vi "Digital Handler.vi"(0 "Variable Index":i32, 1 "Action":T2, 5 "End Tid":dbl, 7 "Value":bool, 9 "Upd freq":T1, 11 "error in (no error)":errorcluster, 12 "Start tid(buff size":dbl) -> (3 "Indexes":i32[](array[numeric]), 6 "Value out":bool, 8 "Digital Waveform":digitalwaveform(waveform)={"t0"=timestamp(0 s since 1904-01-01), "dt"=1.0, "Y"={"transitions"=[], "data"=[]}}, 10 "Values":bool[](array[boolean]), 14 "Numb var":i32, 15 "error out":errorcluster)   [LabVIEW 2010]
uses:
  Action Analog Handler.ctl
  Update frequensies.ctl
  Digital Psudo WF.ctl
  <vilib>/Waveform/DTblOps.llb/DTbl Boolean Array to Digital.vi
panel:
  out "Time Stamp":timestamp
  # "OBS, \nBruk Value som oppdaterings frekvens \nunder reg new var."
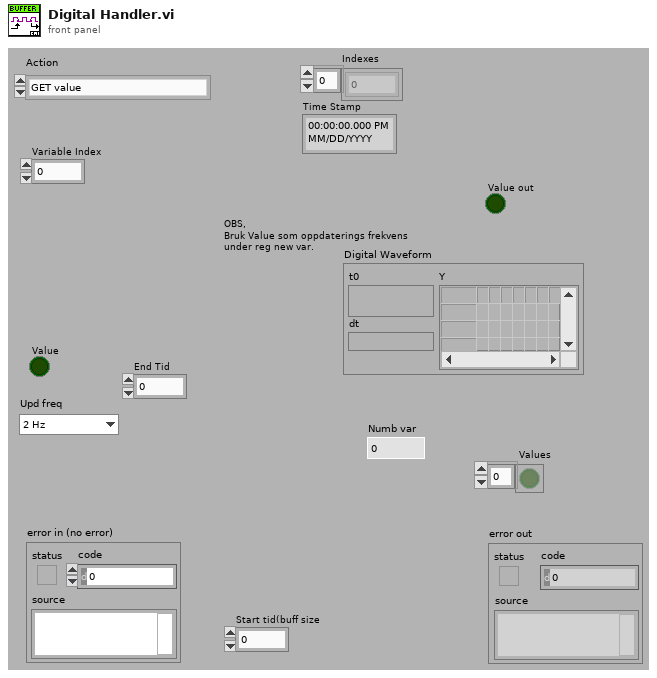
[diagram p1: front panel]
types:
  T1 = typedef "Update frequensies.ctl" = enum16{"2 Hz", "1 Hz", "0.1 Hz"}
  T2 = typedef "Action Analog Handler.ctl" = enum16{"GET value", "GET Single Frequenzy", "GET All Values", "GET Waveform", "Get Numb Var", "SET Value", "START Buffer", "REG Variable", "BUF size(total antal sekund)", "PULS", "Get a Value at time"}
  T3 = typedef "Digital Psudo WF.ctl" = cluster{"\ndata":bool[], "Index":i32, "Upd freq":T1, "Last index time":dbl, "Rounded":bool}
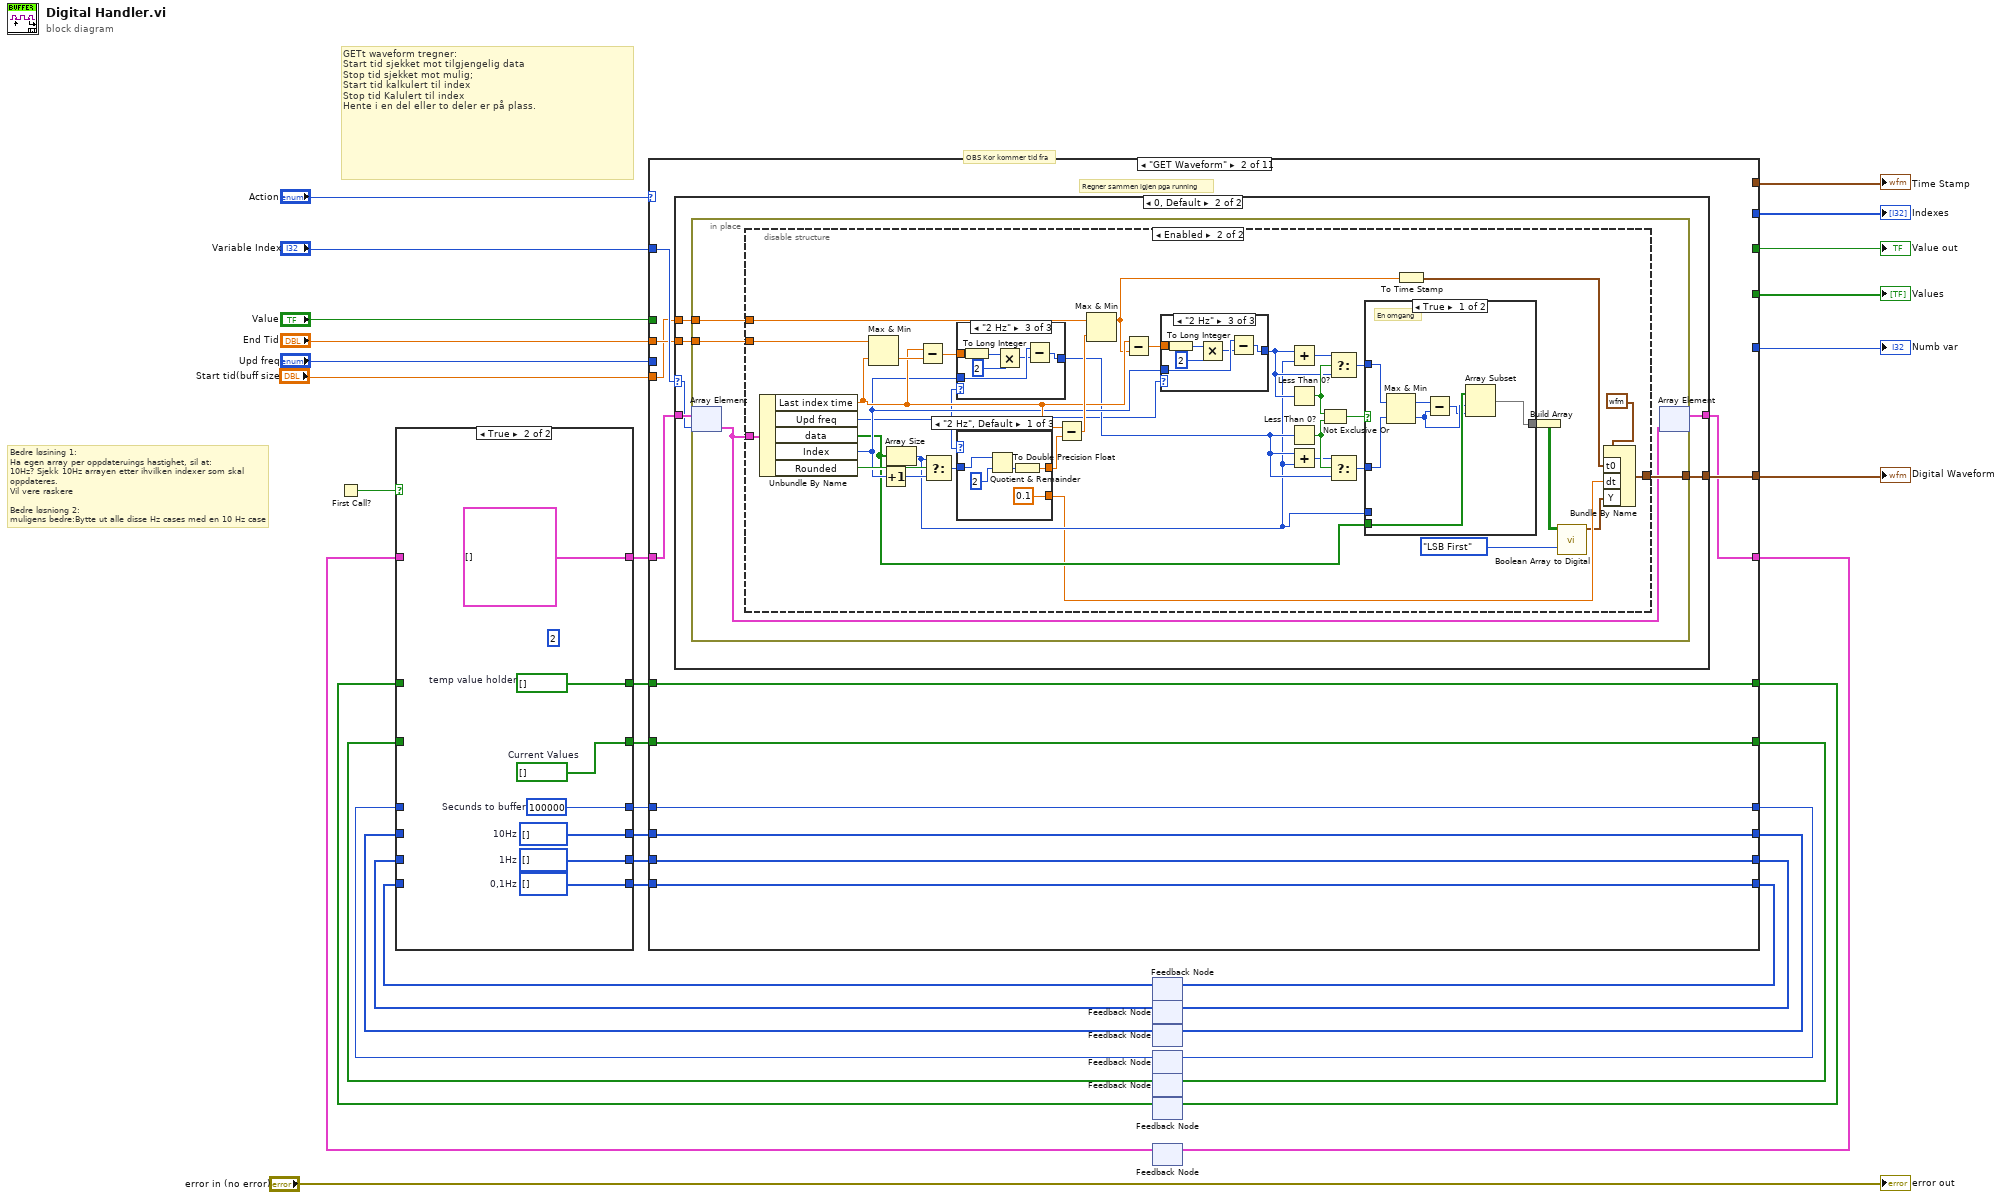
[diagram p0: block diagram]
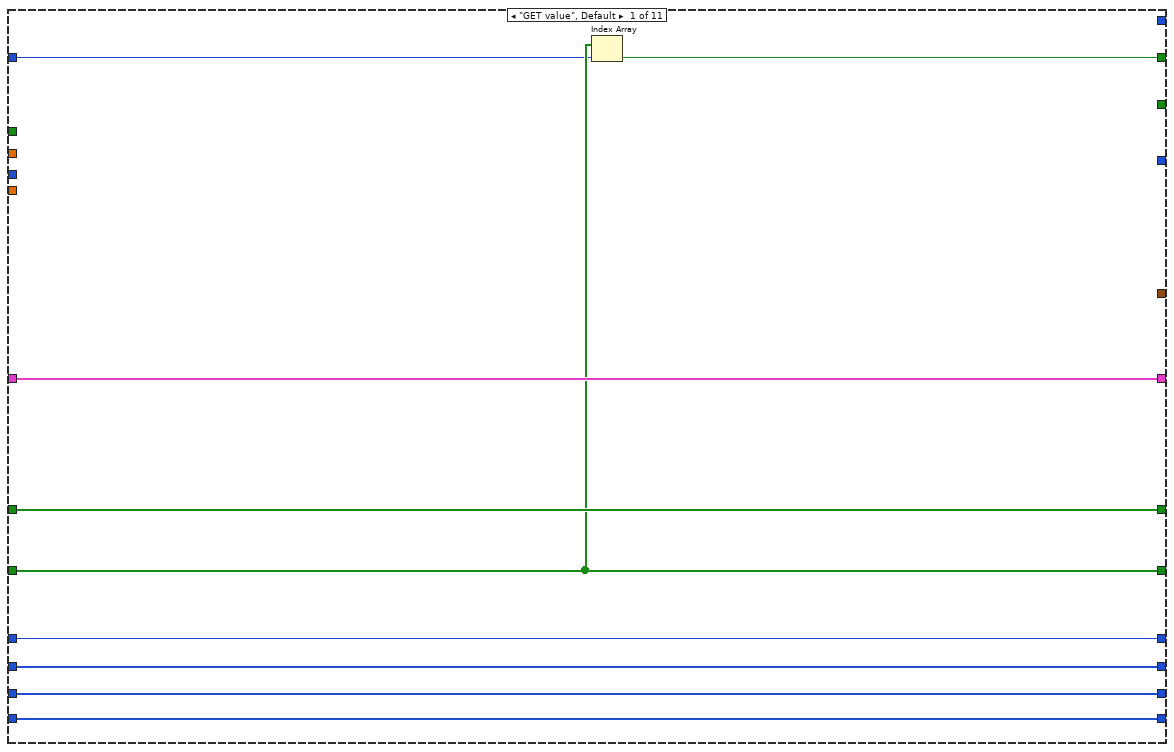
[diagram p3: hidden frame]
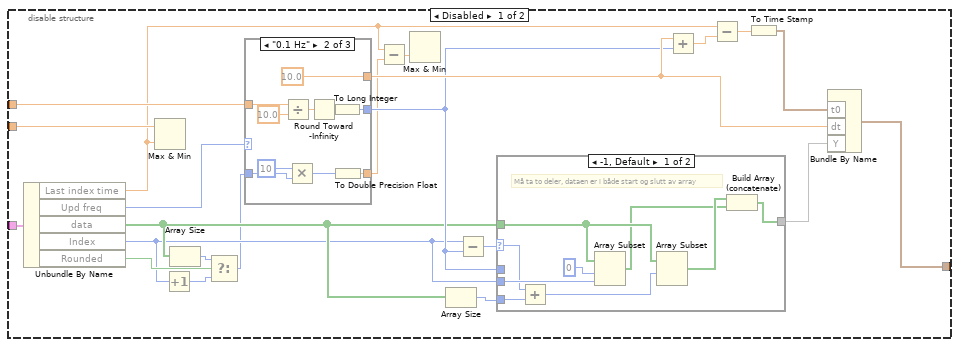
[diagram p5: hidden frame]
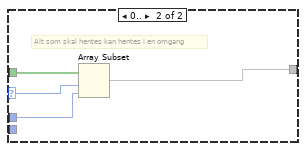
[diagram p6: hidden frame]
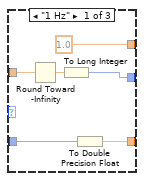
[diagram p7: hidden frame]
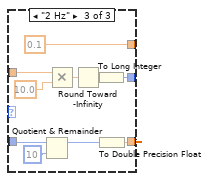
[diagram p8: hidden frame]
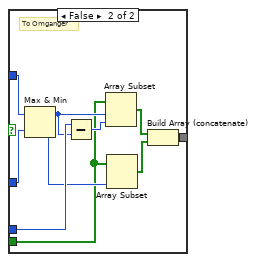
[diagram p9: hidden frame]
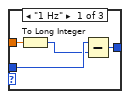
[diagram p10: hidden frame]
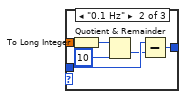
[diagram p11: hidden frame]
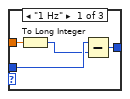
[diagram p12: hidden frame]
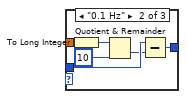
[diagram p13: hidden frame]
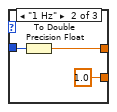
[diagram p14: hidden frame]
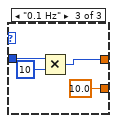
[diagram p15: hidden frame]
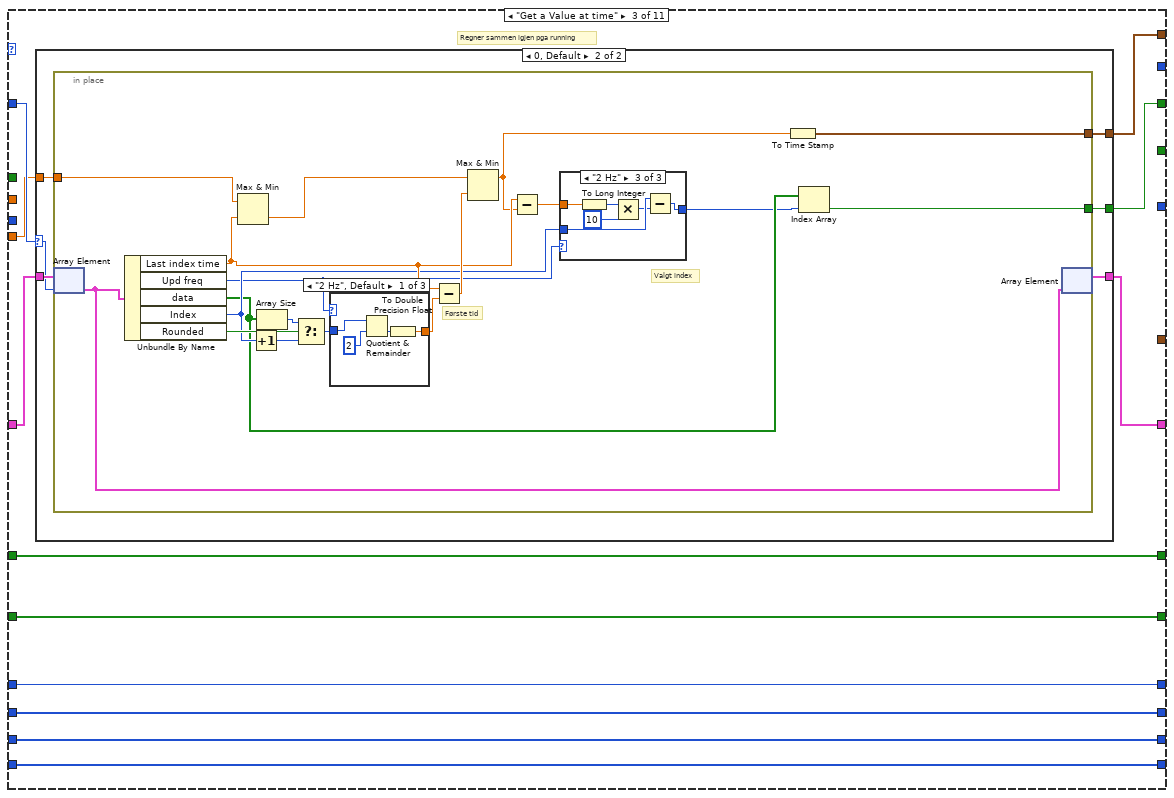
[diagram p16: hidden frame]
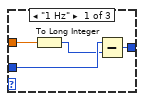
[diagram p18: hidden frame]
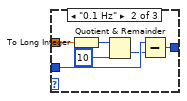
[diagram p19: hidden frame]
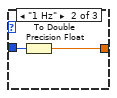
[diagram p20: hidden frame]
diagram:
  # "GETt waveform tregner:\nStart tid sjekket mot tilgjengelig data\nStop tid sjekket mot mulig;\nStart tid kalkulert til index\nStop tid Kalulert til index\nHente i en del eller to deler er på plass."
  # "OBS Kor kommer tid fra"
  # "Bedre løsining 1:\nHa egen array per oppdateruings hastighet, sil at:\n10Hz? Sjekk 10Hz arrayen etter ihvilken indexer som skal oppdateres.\nVil vere raskere\n\nBedre løsniong 2:\nmuligens bedre:Bytte ut alle disse Hz cases med en 10 Hz case"
  n1 = First Call?() -> (First Call?: T/F=w32:bool)
  n2 = feedback #1() -> (w9:i32[])  [unwired: 1 in]
  n3 = feedback #2() -> (w10:i32[])  [unwired: 1 in]
  n4 = feedback #3() -> (w11:i32[])  [unwired: 1 in]
  n5 = feedback #4() -> (w8:i32)  [unwired: 1 in]
  n6 = feedback #5() -> (w25:bool[])  [unwired: 1 in]
  n7 = feedback #6() -> (w26:bool[])  [unwired: 1 in]
  n8 = feedback #7() -> (w33:T3[])  [unwired: 1 in]
  n9 = case shown="True" w32 {
    tunnel: w33 -> [w42 _]
    tunnel: [w42 T3[] []] -> w2
    tunnel: [w41 w49] -> w30
    tunnel: [w40 w48] -> w29
    tunnel: w26 -> [w41 _]
    tunnel: w25 -> [w40 _]
    tunnel: [w36 w47] -> w23
    tunnel: [w39 w46] -> w17
    tunnel: [w38 w45] -> w14
    tunnel: [w37 w44] -> w12
    tunnel: w11 -> [w39 _]
    tunnel: w10 -> [w38 _]
    tunnel: w9 -> [w37 _]
    tunnel: w8 -> [w36 _]
    frame False {
    }
    frame True {
      (unwired) u8 2 ("ValDigital - Status value(0 F, 1 T, 2 NA)")
      w44 = i32[] []  # 0,1Hz
      w45 = i32[] []  # 1Hz
      w46 = i32[] []  # 10Hz
      w47 = 100000  # Secunds to buffer
      w48 = bool[] []  # Current Values
      w49 = bool[] []  # temp value holder
    }
  }
  n10 = case shown="\"GET Waveform\"" "Action" {
    tunnel: [w58 w62 w242 w307 w317 w326 w341 w388 w414 w442 w506] -> w31
    tunnel: w2 -> [w58 w63 w243 w307 w317 w326 w340 w388 w414 w447 w509]
    tunnel: w30 -> [w57 w70 w249 w300 w314 w325 w338 w389 w416 w424 w508]
    tunnel: w29 -> [w56 w69 w248 w306 w316 w324 w336 w395 w410 w443 w507]
    tunnel: [w57 w70 w249 w300 w313 w325 w339 w389 w416 w441 w505] -> w27
    tunnel: [w56 w69 w248 w306 w316 w324 w337 w396 w410 w440 w504] -> w28
    tunnel: [w53 w60 w241 w305 w315 w320 w335 w394 w415 w421 w510] -> w24
    tunnel: w23 -> [w53 w60 w241 w305 w315 _ w335 w394 w415 w421 w510]
    tunnel: "Variable Index" -> [w54 w64 w244 _ w311 _ _ _ _ w423 w503]
    tunnel: "Value" -> [_ _ _ _ w312 _ _ _ _ _ _]
    tunnel: [w55 _ w239 _ _ _ _ _ _ _ _] -> w20
    tunnel: [_ _ _ _ _ _ w329 w386 w410 _ _] -> w19
    tunnel: [_ _ _ w304 _ _ w330 w387 _ _ _] -> w18
    tunnel: w17 -> [w52 w68 w247 w303 w310 w323 w332 w391 w413 w436 w502]
    tunnel: [w52 w68 w247 w303 w310 w323 w332 w391 w413 w430 w502] -> w16
    tunnel: [w51 w67 w246 w302 w309 w322 w334 w393 w412 w427 w501] -> w15
    tunnel: w14 -> [w51 w67 w246 w302 w309 w322 w334 w393 w412 w435 w501]
    tunnel: [w50 w66 w245 w301 w308 w321 w333 w392 w411 w425 w500] -> w13
    tunnel: w12 -> [w50 w66 w245 w301 w308 w321 w333 w392 w411 w434 w500]
    tunnel: [_ w65 _ _ _ _ _ _ _ _ _] -> w1
    tunnel: "Upd freq" -> [_ _ _ _ _ _ w331 w390 _ w418 _]
    tunnel: [_ _ _ _ _ _ w328 w385 w409 _ _] -> w6
    tunnel: "End Tid" -> [_ w61 _ _ _ _ _ _ _ _ _]
    tunnel: [_ _ w240 _ _ _ _ _ _ _ _] -> w4
    tunnel: "Start tid(buff size" -> [_ w59 w238 _ _ w319 w327 _ _ _ _]
    frame "GET value", Default {
      n11 = Index Array(array=w56, index=w54) -> (element=w55:bool)
    }
    frame "GET Waveform" {
      # "Regner sammen igjen pga running"
      n12 = case shown="0, Default" w64 {
        selector: w64 -> [_ w74]
        tunnel: w63 -> [w71 w75]
        tunnel: w59 -> [_ w77]
        tunnel: [_ w76] -> w65
        tunnel: [w71 w73] -> w62
        tunnel: w61 -> [_ w72]
        frame ..-1 {
        }
        frame 0, Default {
          n13 = in-place {
            in-place-border: w77 -> [w79]
            in-place-border: [w81] -> w76
            in-place-border: w72 -> [w78]
            n14 = in-place-array #8(w75, w74) -> (w80:T3)
            n15 = disable-structure shown="Enabled" {
              disable-tunnel: [w94 w176] -> w81
              disable-tunnel: w80 -> [w93 w175]
              disable-tunnel: w79 -> [w87 w168]
              disable-tunnel: w78 -> [w86 w171]
              frame Disabled {
                n16 = Unbundle By Name(w93) -> ("Last index time"=w84:dbl, "Upd freq"=w103:T1, "data"=w91:bool[], "Index"=w90:i32, "Rounded"=w92:bool)
                n17 = Max & Min(x=w86, y=w84) -> ()  [unwired: 2 out]
                n18 = Increment(x=w90) -> (x+1=w89:i32)
                n19 = Array Size(array=w91) -> (size(s)=w88:i32)
                n20 = Select(t=w88, s=w92, f=w89) -> (s? t:f=w85:i32)
                n21 = case shown="\"0.1 Hz\"" w103 {
                  tunnel: w87 -> [w121 w131 w141]
                  tunnel: [w120 w130 w140] -> w98
                  tunnel: [1.0 ("y") 10.0 ("y") 0.1 ("y")] -> w99
                  tunnel: w85 -> [w118 w126 w136]
                  tunnel: [w117 w123 w133] -> w83
                  frame "1 Hz" {
                    n22 = Round Toward -Infinity(1:w121) -> (0:w122:dbl)
                    n23 = To Long Integer(number=w122) -> (32bit integer=w120:i32)
                    n24 = To Double Precision Float(number=w118) -> (double precision float=w117:dbl)
                  }
                  frame "0.1 Hz" {
                    n25 = Divide(x=w131, y=10.0) -> (x/y=w129:dbl)
                    n26 = Multiply(x=10, y=w126) -> (x*y=w124:i32)
                    n27 = Round Toward -Infinity(1:w129) -> (0:w132:dbl)
                    n28 = To Long Integer(number=w132) -> (32bit integer=w130:i32)
                    n29 = To Double Precision Float(number=w124) -> (double precision float=w123:dbl)
                  }
                  frame "2 Hz" {
                    n30 = Quotient & Remainder(x=w136, y=10) -> (x-y*floor(x/y)=w134:i32)  [unwired: 1 out]
                    n31 = Multiply(x=w141, y=10.0) -> (x*y=w139:dbl)
                    n32 = Round Toward -Infinity(1:w139) -> (0:w142:dbl)
                    n33 = To Long Integer(number=w142) -> (32bit integer=w140:i32)
                    n34 = To Double Precision Float(number=w134) -> (double precision float=w133:dbl)
                  }
                }
                n35 = Subtract(x=w84, y=w83) -> (x-y=w82:dbl)
                n36 = Max & Min(y=w82) -> ()  [unwired: 1 in, 2 out]
                n37 = Array Size(array=w91) -> (size(s)=w101:i32)
                n38 = Subtract(x=w90, y=w98) -> (x-y=w102:i32)
                n39 = case shown="-1, Default" w102 {
                  selector: w102 -> [w109 w115]
                  tunnel: w91 -> [w108 w116]
                  tunnel: w98 -> [_ w114]
                  tunnel: [w104 w113] -> w100
                  tunnel: w90 -> [w111 _]
                  tunnel: w101 -> [w110 _]
                  frame -1, Default {
                    # "Må ta to deler, dataen er i både start og slutt av array"
                    n40 = Add(x=w109, y=w110) -> (x+y=w107:i32)
                    n41 = Array Subset(array=w108, index=0, length=w111) -> (w105:bool[])
                    n42 = Array Subset(array=w108, index=w107) -> (w106:bool[])  [unwired: 1 in]
                    n43 = Build Array (concatenate)(w106, w105) -> (w104:bool[])
                  }
                  frame 0.. {
                    # "Alt som skal hentes kan hentes i en omgang"
                    n44 = Array Subset(array=w116, index=w115, length=w114) -> (w113:bool[])
                  }
                }
                n45 = Add(x=w99, y=w98) -> (x+y=w97:dbl)
                n46 = Subtract(x=w84, y=w97) -> (x-y=w96:dbl)
                n47 = To Time Stamp(1:w96) -> (0:w95:timestamp)
                n48 = Bundle By Name("t0"=w95, "dt"=w99, "Y"=w100) -> (w94:waveform(u8))  [unwired: 1 in]
              }
              frame Enabled {
                n49 = Unbundle By Name(w175) -> ("Last index time"=w165:dbl, "Upd freq"=w149:T1, "data"=w153:bool[], "Index"=w163:i32, "Rounded"=w174:bool)
                n50 = Max & Min(x=w171, y=w165) -> (min(x,y)=w167:dbl)  [unwired: 1 out]
                n51 = Increment(x=w163) -> (x+1=w173:i32)
                n52 = Array Size(array=w153) -> (size(s)=w152:i32)
                n53 = Subtract(x=w165, y=w167) -> (x-y=w166:dbl)
                n54 = Select(t=w152, s=w174, f=w173) -> (s? t:f=w172:i32)
                n55 = case shown="\"2 Hz\"" w149 {
                  tunnel: w163 -> [w212 w218 w224]
                  tunnel: w166 -> [w213 w219 w225]
                  tunnel: [w210 w216 w222] -> w160
                  frame "1 Hz" {
                    n56 = To Long Integer(number=w213) -> (32bit integer=w211:i32)
                    n57 = Subtract(x=w212, y=w211) -> (x-y=w210:i32)
                  }
                  frame "0.1 Hz" {
                    n58 = To Long Integer(number=w219) -> (32bit integer=w217:i32)
                    n59 = Quotient & Remainder(x=w217, y=10) -> (floor(x/y)=w215:i32)  [unwired: 1 out]
                    n60 = Subtract(x=w218, y=w215) -> (x-y=w216:i32)
                  }
                  frame "2 Hz" {
                    n61 = To Long Integer(number=w225) -> (32bit integer=w223:i32)
                    n62 = Multiply(x=w223, y=2) -> (x*y=w221:i32)
                    n63 = Subtract(x=w224, y=w221) -> (x-y=w222:i32)
                  }
                }
                n64 = case shown="\"2 Hz\", Default" w149 {
                  tunnel: w172 -> [w230 w233 w237]
                  tunnel: [w229 w232 w235] -> w170
                  tunnel: [0.1 ("dt") 1.0 ("dt") 10.0 ("dt")] -> w145
                  frame "2 Hz", Default {
                    n65 = Quotient & Remainder(x=w230, y=2 ("x")) -> (floor(x/y)=w228:i32)  [unwired: 1 out]
                    n66 = To Double Precision Float(number=w228) -> (double precision float=w229:dbl)
                  }
                  frame "1 Hz" {
                    n67 = To Double Precision Float(number=w233) -> (double precision float=w232:dbl)
                  }
                  frame "0.1 Hz" {
                    n68 = Multiply(x=w237, y=10) -> (x*y=w235:i32)
                  }
                }
                n69 = Subtract(x=w165, y=w170) -> (x-y=w169:dbl)
                n70 = Max & Min(x=w168, y=w169) -> (max(x,y)=w151:dbl)  [unwired: 1 out]
                n71 = Subtract(x=w165, y=w151) -> (x-y=w164:dbl)
                n72 = case shown="\"2 Hz\"" w149 {
                  tunnel: w163 -> [w196 w202 w208]
                  tunnel: w164 -> [w197 w203 w209]
                  tunnel: [w194 w200 w206] -> w157
                  frame "1 Hz" {
                    n73 = To Long Integer(number=w197) -> (32bit integer=w195:i32)
                    n74 = Subtract(x=w196, y=w195) -> (x-y=w194:i32)
                  }
                  frame "0.1 Hz" {
                    n75 = To Long Integer(number=w203) -> (32bit integer=w201:i32)
                    n76 = Quotient & Remainder(x=w201, y=10) -> (floor(x/y)=w199:i32)  [unwired: 1 out]
                    n77 = Subtract(x=w202, y=w199) -> (x-y=w200:i32)
                  }
                  frame "2 Hz" {
                    n78 = To Long Integer(number=w209) -> (32bit integer=w207:i32)
                    n79 = Multiply(x=w207, y=2) -> (x*y=w205:i32)
                    n80 = Subtract(x=w208, y=w205) -> (x-y=w206:i32)
                  }
                }
                n81 = Add(x=w157, y=w152) -> (x+y=w158:i32)
                n82 = Less Than 0?(x=w157) -> (x < 0?=w162:bool)
                n83 = Less Than 0?(x=w160) -> (x < 0?=w161:bool)
                n84 = Add(x=w160, y=w152) -> (x+y=w159:i32)
                n85 = Not Exclusive Or(1:w161, 2:w162) -> (0:w156:bool)
                n86 = Select(t=w158, s=w162, f=w157) -> (s? t:f=w155:i32)
                n87 = Select(t=w159, s=w161, f=w160) -> (s? t:f=w154:i32)
                n88 = case shown="True" w156 {
                  tunnel: w155 -> [w183 w193]
                  tunnel: w154 -> [w182 w192]
                  tunnel: w153 -> [w180 w187]
                  tunnel: [w177 w184] -> w147
                  tunnel: w152 -> [_ w191]
                  frame True {
                    # "En omgang"
                    n89 = Max & Min(x=w183, y=w182) -> (max(x,y)=w181:i32, min(x,y)=w179:i32)
                    n90 = Subtract(x=w181, y=w179) -> (x-y=w178:i32)
                    n91 = Array Subset(array=w180, index=w179, length=w178) -> (w177:bool[])
                  }
                  frame False {
                    # "To Omganger"
                    n92 = Max & Min(x=w193, y=w192) -> (max(x,y)=w190:i32, min(x,y)=w188:i32)
                    n93 = Subtract(x=w191, y=w190) -> (x-y=w189:i32)
                    n94 = Array Subset(array=w187, index=w190, length=w189) -> (w186:bool[])
                    n95 = Array Subset(array=w187, length=w188) -> (w185:bool[])  [unwired: 1 in]
                    n96 = Build Array (concatenate)(w186, w185) -> (w184:bool[])
                  }
                }
                n97 = To Time Stamp(1:w151) -> (0:w150:timestamp)
                n98 = Build Array(w147) -> (w146:bool[][])
                n99 = call-poly <vilib>:"Boolean Array to Digital.vi"("mode"=enum16{"LSB First", "MSB First"}."LSB First", "boolean array"=w146) -> ("digital data"=w143:digitaldata)  [unwired: 8 in, 1 out]
                n100 = Bundle By Name(cluster=digitalwaveform {"t0"=timestamp(0 s since 1904-01-01), "dt"=1.0, "Y"={"transitions"=[], "data"=[]}} ("Digital Waveform"), "t0"=w150, "dt"=w145, "Y"=w143) -> (w176:digitalwaveform)
              }
            }
            n101 = in-place-array #8(w80) -> (w73:T3[])  [unwired: 1 out]
          }
        }
      }
    }
    frame "Get a Value at time" {
      # "Regner sammen igjen pga running"
      n102 = case shown="0, Default" w244 {
        selector: w244 -> [_ w254]
        tunnel: w243 -> [w250 w255]
        tunnel: w238 -> [_ w256]
        tunnel: [w250 w253] -> w242
        tunnel: [_ w252] -> w240
        tunnel: [_ w251] -> w239
        frame ..-1 {
        }
        frame 0, Default {
          n103 = in-place {
            in-place-border: w256 -> [w274]
            in-place-border: [w259] -> w252
            in-place-border: [w258] -> w251
            # "Valgt index"
            # "Første tid"
            n104 = in-place-array #9(w255, w254) -> (w257:T3)
            n105 = Unbundle By Name(w257) -> ("Last index time"=w268:dbl, "Upd freq"=w263:T1, "data"=w261:bool[], "Index"=w266:i32, "Rounded"=w273:bool)
            n106 = Max & Min(x=w274, y=w268) -> (min(x,y)=w262:dbl)  [unwired: 1 out]
            n107 = Increment(x=w266) -> (x+1=w272:i32)
            n108 = Array Size(array=w261) -> (size(s)=w265:i32)
            n109 = Select(t=w265, s=w273, f=w272) -> (s? t:f=w271:i32)
            n110 = case shown="\"2 Hz\", Default" w263 {
              tunnel: w271 -> [w294 w296 w299]
              tunnel: [w293 w295 w297] -> w270
              frame "2 Hz", Default {
                n111 = Quotient & Remainder(x=w294, y=2 ("x")) -> (floor(x/y)=w292:i32)  [unwired: 1 out]
                n112 = To Double Precision Float(number=w292) -> (double precision float=w293:dbl)
              }
              frame "1 Hz" {
                n113 = To Double Precision Float(number=w296) -> (double precision float=w295:dbl)
              }
              frame "0.1 Hz" {
                n114 = Multiply(x=w299, y=10) -> (x*y=w297:i32)
              }
            }
            n115 = Subtract(x=w268, y=w270) -> (x-y=w269:dbl)
            n116 = Max & Min(x=w262, y=w269) -> (max(x,y)=w264:dbl)  [unwired: 1 out]
            n117 = Subtract(x=w268, y=w264) -> (x-y=w267:dbl)
            n118 = case shown="\"2 Hz\"" w263 {
              tunnel: w266 -> [w277 w283 w289]
              tunnel: w267 -> [w278 w284 w290]
              tunnel: [w275 w281 w287] -> w260
              frame "1 Hz" {
                n119 = To Long Integer(number=w278) -> (32bit integer=w276:i32)
                n120 = Subtract(x=w277, y=w276) -> (x-y=w275:i32)
              }
              frame "0.1 Hz" {
                n121 = To Long Integer(number=w284) -> (32bit integer=w282:i32)
                n122 = Quotient & Remainder(x=w282, y=10) -> (floor(x/y)=w280:i32)  [unwired: 1 out]
                n123 = Subtract(x=w283, y=w280) -> (x-y=w281:i32)
              }
              frame "2 Hz" {
                n124 = To Long Integer(number=w290) -> (32bit integer=w288:i32)
                n125 = Multiply(x=w288, y=10) -> (x*y=w286:i32)
                n126 = Subtract(x=w289, y=w286) -> (x-y=w287:i32)
              }
            }
            n127 = To Time Stamp(1:w264) -> (0:w259:timestamp)
            n128 = Index Array(array=w261, index=w260) -> (element=w258:bool)
            n129 = in-place-array #9(w257) -> (w253:T3[])  [unwired: 1 out]
          }
        }
      }
    }
    frame "Get Numb Var" {
      n130 = Array Size(array=w300) -> (size(s)=w304:i32)
    }
    frame "SET Value" {
      n131 = in-place {
        in-place-border: w312 -> [w318]
        n132 = in-place-array #10(w314, w311) -> ()  [unwired: 1 out]
        n133 = in-place-array #10(w318) -> (w313:bool[])  [unwired: 1 out]
      }
    }
    frame "BUF size(total antal sekund)" {
      n134 = To Long Integer(number=w319) -> (32bit integer=w320:i32)
    }
    frame "PULS" {
      n135 = case shown="\"0.1 Hz\"" w331 {
        tunnel: w332 -> [_ w344 _]
        tunnel: w334 -> [_ _ w345]
        tunnel: w333 -> [w343 _ _]
        tunnel: [w343 w344 w345] -> w328
        frame "0.1 Hz" {
        }
        frame "2 Hz" {
        }
        frame "1 Hz" {
        }
      }
      n136 = Empty Array?(array=w328) -> (empty?=w342:bool)
      n137 = case shown="False" w342 {
        tunnel: [w350 w384] -> w341
        tunnel: w340 -> [w352 w384]
        tunnel: [w349 w383] -> w339
        tunnel: w338 -> [w353 w383]
        tunnel: [w348 w382] -> w337
        tunnel: w336 -> [w354 w382]
        tunnel: w328 -> [w351 _]
        tunnel: w327 -> [w347 _]
        tunnel: [w346 _] -> w329
        frame False {
          n138 = for {
            tunnel: w351 -> [w358] mode=indexing
            shift-right: [w357] -> w350
            shift-left: w352 -> [w359]
            shift-right: [w360] -> w349
            shift-left: w353 -> [w361]
            shift-right: [w362] -> w348
            shift-left: w354 -> [w363]
            tunnel: w347 -> [w356]
            tunnel: [w355] -> w346 mode=indexing
            n139 = in-place {
              in-place-border: w356 -> [w366]
              in-place-border: [w365] -> w355
              n140 = in-place-array #11(w359, w358) -> (w368:T3)
              n141 = in-place-array #12(w361, w358) -> (w365:bool)
              n142 = in-place-array #13(w363, w358) -> ()  [unwired: 1 out]
              n143 = in-place {
                in-place-border: w365 -> [w373]
                in-place-border: w366 -> [w372]
                # "Antall skal ikke endre seg"
                n144 = in-place-cluster #14(w368) -> ("data"=w376:bool[], "Index"=w374:i32, "Rounded"=w371:bool)  [unwired: 1 out]
                n145 = in-place {
                  in-place-border: w373 -> [w381]
                  n146 = in-place-array #15(w376, w374) -> ()  [unwired: 1 out]
                  n147 = in-place-array #15(w381) -> (w375:bool[])  [unwired: 1 out]
                }
                n148 = Array Size(array=w376) -> (size(s)=w380:i32)
                n149 = Increment(x=w374) -> (x+1=w379:i32)
                n150 = Greater Or Equal?(x=w379, y=w380) -> (x >= y?=w370:bool)
                n151 = Select(t=0, s=w370, f=w379) -> (s? t:f=w377:i32)
                n152 = Or(x=w370, y=w371) -> (x .or. y?=w369:bool)
                n153 = in-place-cluster #14("Last index time"=w372, "data"=w375, "Index"=w377, "Rounded"=w369) -> (w367:T3)
              }
              n154 = in-place-array #11(w367) -> (w357:T3[])  [unwired: 1 out]
              n155 = in-place-array #12(FALSE) -> (w360:bool[])  [unwired: 1 out]
              n156 = in-place-array #13(w365) -> (w362:bool[])  [unwired: 1 out]
            }
          }
        }
        frame True {
          # "Ingen 10 Hzere"
        }
      }
      n157 = Array Size(array=w329) -> (size(s)=w330:i32)
    }
    frame "GET Single Frequenzy" {
      n158 = case shown="\"0.1 Hz\"" w390 {
        tunnel: w391 -> [_ w399 _]
        tunnel: w393 -> [_ _ w400]
        tunnel: w392 -> [w398 _ _]
        tunnel: [w398 w399 w400] -> w385
        frame "0.1 Hz" {
        }
        frame "2 Hz" {
        }
        frame "1 Hz" {
        }
      }
      n159 = Empty Array?(array=w385) -> (empty?=w397:bool)
      n160 = case shown="False" w397 {
        tunnel: [w403 w408] -> w396
        tunnel: w395 -> [w404 w408]
        tunnel: w385 -> [w402 _]
        tunnel: [w401 _] -> w386
        frame False {
          n161 = for {
            shift-right: [w406] -> w403
            shift-left: w404 -> [w406]
            tunnel: w402 -> [w407] mode=indexing
            tunnel: [w405] -> w401 mode=indexing
            n162 = Index Array(array=w406, index=w407) -> (element=w405:bool)
          }
        }
        frame True {
        }
      }
      n163 = Array Size(array=w386) -> (size(s)=w387:i32)
    }
    frame "GET All Values" {
      n164 = for {
        tunnel: w410 -> [_] mode=indexing
        tunnel: [w417] -> w409 mode=indexing
        i -> [w417]
      }
    }
    frame "REG Variable" {
      # "Fjerner den nye, om den ligger i en av listene"
      n165 = To Long Integer(number=w423) -> (32bit integer=w422:i32)
      n166 = Increment(x=w422) -> (x+1=w438:i32)
      n167 = Search 1D Array(1D array=w434, element=w422) -> (index of element=w433:i32)  [unwired: 1 in]
      n168 = Array Size(array=w424) -> (size(s)=w439:i32)
      n169 = Subtract(x=w438, y=w439) -> (x-y=w437:i32)
      n170 = Delete From Array(array=w434, index=w433) -> (array with subset deleted=w426:i32[])  [unwired: 1 in, 1 out]
      n171 = Search 1D Array(1D array=w435, element=w422) -> (index of element=w431:i32)  [unwired: 1 in]
      n172 = case shown="\"2 Hz\"" w418 {
        selector: w418 -> [w448 w452 w456]
        tunnel: w421 -> [w451 w455 w457]
        tunnel: [w449 w453 w457] -> w420
        tunnel: [w448 w452 w456] -> w419
        frame "2 Hz" {
          n173 = Multiply(x=w451, y=2) -> (x*y=w449:i32)
        }
        frame "0.1 Hz" {
          n174 = Quotient & Remainder(x=w455, y=10) -> (floor(x/y)=w453:i32)  [unwired: 1 out]
        }
        frame "1 Hz" {
        }
      }
      n175 = Delete From Array(array=w435, index=w431) -> (array with subset deleted=w428:i32[])  [unwired: 1 in, 1 out]
      n176 = case shown="1, Default" w437 {
        selector: w437 -> [_ w485]
        tunnel: w447 -> [w475 w492]
        tunnel: [w475 w491] -> w446
        tunnel: [w474 w490] -> w445
        tunnel: w424 -> [w474 w488]
        tunnel: [w473 w489] -> w444
        tunnel: w443 -> [w473 w487]
        tunnel: w420 -> [_ w480]
        tunnel: w419 -> [_ w479]
        frame 0 {
        }
        frame 1, Default {
          w478 = FALSE
          n177 = Initialize Array(FALSE, w480) -> (w482:bool[])
          n178 = Bundle By Name(cluster=T3 {"\ndata"=[], "Index"=0, "Upd freq"=enum."2 Hz", "Last index time"=0.0, "Rounded"=FALSE} ("Cluster"), "data"=w482, "Upd freq"=w479) -> (w481:T3)
          n179 = Initialize Array(w481, w485) -> (w486:T3[])
          n180 = Initialize Array(w478, w485) -> (w484:bool[])
          n181 = Initialize Array(w478, w485) -> (w483:bool[])
          n182 = Build Array (concatenate)(w492, w486) -> (w491:T3[])
          n183 = Build Array (concatenate)(w488, w484) -> (w490:bool[])
          n184 = Build Array (concatenate)(w487, w483) -> (w489:bool[])
        }
      }
      n185 = Search 1D Array(1D array=w436, element=w422) -> (index of element=w432:i32)  [unwired: 1 in]
      n186 = Delete From Array(array=w436, index=w432) -> (array with subset deleted=w429:i32[])  [unwired: 1 in, 1 out]
      n187 = case shown="\"2 Hz\"" w418 {
        tunnel: [w462 w464 w472] -> w430
        tunnel: w429 -> [w462 w467 w472]
        tunnel: w428 -> [w461 w466 w471]
        tunnel: [w461 w466 w469] -> w427
        tunnel: w426 -> [w460 w465 w470]
        tunnel: [w459 w465 w470] -> w425
        tunnel: w422 -> [w458 w463 w468]
        frame "0.1 Hz" {
          n188 = Build Array (concatenate)(w460, w458) -> (w459:i32[])
        }
        frame "2 Hz" {
          n189 = Build Array (concatenate)(w467, w463) -> (w464:i32[])
        }
        frame "1 Hz" {
          n190 = Build Array (concatenate)(w471, w468) -> (w469:i32[])
        }
      }
      n191 = in-place {
        in-place-border: w420 -> [w496]
        in-place-border: w419 -> [w495]
        w493 = FALSE
        (unwired) nan ("element")
        n192 = in-place-array #16(w446, w422) -> ()  [unwired: 1 out]
        n193 = in-place-array #17(w445, w422) -> ()  [unwired: 1 out]
        n194 = in-place-array #18(w444, w422) -> ()  [unwired: 1 out]
        n195 = Initialize Array(FALSE, w496) -> (w498:bool[])
        n196 = Bundle By Name(cluster=T3 {"\ndata"=[], "Index"=0, "Upd freq"=enum."2 Hz", "Last index time"=0.0, "Rounded"=FALSE} ("Cluster"), "data"=w498, "Upd freq"=w495) -> (w497:T3)
        n197 = in-place-array #16(w497) -> (w442:T3[])  [unwired: 1 out]
        n198 = in-place-array #17(w493) -> (w441:bool[])  [unwired: 1 out]
        n199 = in-place-array #18(w493) -> (w440:bool[])  [unwired: 1 out]
      }
    }
    frame "START Buffer" {
      n200 = in-place {
        w511 = FALSE
        n201 = in-place-array #19(w509, w503) -> (w516:T3)
        n202 = in-place-array #20(w508, w503) -> ()  [unwired: 1 out]
        n203 = in-place-array #21(w507, w503) -> ()  [unwired: 1 out]
        n204 = Unbundle By Name(w516) -> ("data"=w515:bool[])
        n205 = Array Size(array=w515) -> (size(s)=w514:i32)
        n206 = Initialize Array(w511, w514) -> (w517:bool[])
        n207 = Bundle By Name(cluster=T3 {"\ndata"=[], "Index"=0, "Upd freq"=enum."2 Hz", "Last index time"=0.0, "Rounded"=FALSE} ("Cluster"), "data"=w517) -> (w513:T3)
        n208 = in-place-array #19(w513) -> (w506:T3[])  [unwired: 1 out]
        n209 = in-place-array #20(w511) -> (w505:bool[])  [unwired: 1 out]
        n210 = in-place-array #21(w511) -> (w504:bool[])  [unwired: 1 out]
      }
    }
  }
  "Values" <- w19
  "Value out" <- w20
  "Numb var" <- w18
  "Indexes" <- w6
  "Time Stamp" <- w4
  "Digital Waveform" <- w1
  n211 = feedback-in #1(w13) -> ()
  n212 = feedback-in #2(w15) -> ()
  n213 = feedback-in #3(w16) -> ()
  n214 = feedback-in #4(w24) -> ()
  n215 = feedback-in #5(w28) -> ()
  n216 = feedback-in #6(w27) -> ()
  n217 = feedback-in #7(w31) -> ()
  "error out" <- "error in (no error)"
